vi "Main.vi"(7 "sweep rate, /min":dbl=0.2, 8 "sweep to:":dbl=-0.5, 9 "sweep":T3(radio)=enum."time_sweep") -> ()   [LabVIEW 2017] (continued)
                  n2558 = property on="data" class="Arr (strict)"("Value"=w3368) -> ()  [unwired: 2 in, 2 out]
                }
                frame #8 {
                  # "check if voltage \non 2400 SouceMeter 1\nis to be measured"
                  n2559 = property on="data" class="Arr (strict)"() -> ("Value"=w3380:dbl[])  [unwired: 2 in, 2 out]
                  n2560 = local read "2400 1 meas v"() -> (w3379:bool)
                  n2561 = case shown="True" w3379 {
                    tunnel: w3380 -> [w3382 w3393]
                    tunnel: [w3382 w3392] -> w3381
                    frame False {
                      # "we are not measuring 2400 1, voltage (2400_1_v)"
                    }
                    frame True {
                      # "we are  measuring 2400 1, voltage (2400_1_v)"
                      n2562 = local read "2400 1 addr"() -> (w3387:u8)
                      n2563 = Number To Decimal String(number=w3387) -> (decimal integer string=w3386:string)  [unwired: 1 in]
                      n2564 = GPIB Write(0:w3386, 1:":READ?") -> (6:w3391:errorcluster)  [unwired: 3 in, 1 out]
                      n2565 = GPIB Read(0:w3386, 1:3200, 3:w3391) -> (5:w3384:string)  [unwired: 2 in, 2 out]
                      n2566 = String Subset(string=w3384, length (rest)=13) -> (substring=w3383:string)  [unwired: 1 in]
                      n2567 = Fract/Exp String To Number(string=w3383) -> (number=w3389:dbl)  [unwired: 3 in, 1 out]
                      n2568 = Build Array (concatenate)(w3393, w3389) -> (w3392:dbl[])
                    }
                  }
                  n2569 = property on="data" class="Arr (strict)"("Value"=w3381) -> ()  [unwired: 2 in, 2 out]
                }
                frame #9 {
                  # "check if current \non 2400 SouceMeter 1\nis to be measured"
                  n2570 = property on="data" class="Arr (strict)"() -> ("Value"=w3395:dbl[])  [unwired: 2 in, 2 out]
                  n2571 = local read "2400 1 meas i"() -> (w3394:bool)
                  n2572 = case shown="True" w3394 {
                    tunnel: w3395 -> [w3397 w3409]
                    tunnel: [w3397 w3408] -> w3396
                    frame False {
                      # "we are not measuring 2400 1, current (2400_1_i)"
                    }
                    frame True {
                      # "we are  measuring 2400 1, current (2400_1_i)"
                      n2573 = local read "2400 1 addr"() -> (w3403:u8)
                      n2574 = Number To Decimal String(number=w3403) -> (decimal integer string=w3402:string)  [unwired: 1 in]
                      n2575 = GPIB Write(0:w3402, 1:":READ?") -> (6:w3407:errorcluster)  [unwired: 3 in, 1 out]
                      n2576 = GPIB Read(0:w3402, 1:3200, 3:w3407) -> (5:w3400:string)  [unwired: 2 in, 2 out]
                      n2577 = String Subset(string=w3400, offset (0)=14, length (rest)=13) -> (substring=w3399:string)
                      n2578 = Fract/Exp String To Number(string=w3399) -> (number=w3405:dbl)  [unwired: 3 in, 1 out]
                      n2579 = Build Array (concatenate)(w3409, w3405) -> (w3408:dbl[])
                    }
                  }
                  n2580 = property on="data" class="Arr (strict)"("Value"=w3396) -> ()  [unwired: 2 in, 2 out]
                }
                frame #10 {
                  # "check if voltage \non 2400 SouceMeter 2\nis to be measured"
                  n2581 = property on="data" class="Arr (strict)"() -> ("Value"=w3411:dbl[])  [unwired: 2 in, 2 out]
                  n2582 = local read "2400 2 meas v"() -> (w3410:bool)
                  n2583 = case shown="True" w3410 {
                    tunnel: w3411 -> [w3413 w3424]
                    tunnel: [w3413 w3423] -> w3412
                    frame False {
                      # "we are not measuring 2400 2, voltage (2400_2_v)"
                    }
                    frame True {
                      # "we are  measuring 2400 2, voltage (2400_2_v)"
                      n2584 = local read "2400 2 addr"() -> (w3418:u8)
                      n2585 = Number To Decimal String(number=w3418) -> (decimal integer string=w3417:string)  [unwired: 1 in]
                      n2586 = GPIB Write(0:w3417, 1:":READ?") -> (6:w3422:errorcluster)  [unwired: 3 in, 1 out]
                      n2587 = GPIB Read(0:w3417, 1:3200, 3:w3422) -> (5:w3415:string)  [unwired: 2 in, 2 out]
                      n2588 = String Subset(string=w3415, length (rest)=13) -> (substring=w3414:string)  [unwired: 1 in]
                      n2589 = Fract/Exp String To Number(string=w3414) -> (number=w3420:dbl)  [unwired: 3 in, 1 out]
                      n2590 = Build Array (concatenate)(w3424, w3420) -> (w3423:dbl[])
                    }
                  }
                  n2591 = property on="data" class="Arr (strict)"("Value"=w3412) -> ()  [unwired: 2 in, 2 out]
                }
                frame #11 {
                  # "check if current \non 2400 SouceMeter 2\nis to be measured"
                  n2592 = property on="data" class="Arr (strict)"() -> ("Value"=w3426:dbl[])  [unwired: 2 in, 2 out]
                  n2593 = local read "2400 2 meas i"() -> (w3425:bool)
                  n2594 = case shown="True" w3425 {
                    tunnel: w3426 -> [w3428 w3440]
                    tunnel: [w3428 w3439] -> w3427
                    frame False {
                      # "we are not measuring 2400 2, current (2400_2_i)"
                    }
                    frame True {
                      # "we are  measuring 2400 2, current (2400_2_i)"
                      n2595 = local read "2400 2 addr"() -> (w3434:u8)
                      n2596 = Number To Decimal String(number=w3434) -> (decimal integer string=w3433:string)  [unwired: 1 in]
                      n2597 = GPIB Write(0:w3433, 1:":READ?") -> (6:w3438:errorcluster)  [unwired: 3 in, 1 out]
                      n2598 = GPIB Read(0:w3433, 1:3200, 3:w3438) -> (5:w3431:string)  [unwired: 2 in, 2 out]
                      n2599 = String Subset(string=w3431, offset (0)=14, length (rest)=13) -> (substring=w3430:string)
                      n2600 = Fract/Exp String To Number(string=w3430) -> (number=w3436:dbl)  [unwired: 3 in, 1 out]
                      n2601 = Build Array (concatenate)(w3440, w3436) -> (w3439:dbl[])
                    }
                  }
                  n2602 = property on="data" class="Arr (strict)"("Value"=w3427) -> ()  [unwired: 2 in, 2 out]
                }
                frame #12 {
                  # "check if voltage \non 2400 SouceMeter 3\nis to be measured"
                  n2603 = property on="data" class="Arr (strict)"() -> ("Value"=w3442:dbl[])  [unwired: 2 in, 2 out]
                  n2604 = local read "2400 3 meas v"() -> (w3441:bool)
                  n2605 = case shown="True" w3441 {
                    tunnel: w3442 -> [w3444 w3455]
                    tunnel: [w3444 w3454] -> w3443
                    frame False {
                      # "we are not measuring 2400 3, voltage (2400_3_v)"
                    }
                    frame True {
                      # "we are  measuring 2400 3, voltage (2400_3_v)"
                      n2606 = local read "2400 3 addr"() -> (w3449:u8)
                      n2607 = Number To Decimal String(number=w3449) -> (decimal integer string=w3448:string)  [unwired: 1 in]
                      n2608 = GPIB Write(0:w3448, 1:":READ?") -> (6:w3453:errorcluster)  [unwired: 3 in, 1 out]
                      n2609 = GPIB Read(0:w3448, 1:3200, 3:w3453) -> (5:w3446:string)  [unwired: 2 in, 2 out]
                      n2610 = String Subset(string=w3446, length (rest)=13) -> (substring=w3445:string)  [unwired: 1 in]
                      n2611 = Fract/Exp String To Number(string=w3445) -> (number=w3451:dbl)  [unwired: 3 in, 1 out]
                      n2612 = Build Array (concatenate)(w3455, w3451) -> (w3454:dbl[])
                    }
                  }
                  n2613 = property on="data" class="Arr (strict)"("Value"=w3443) -> ()  [unwired: 2 in, 2 out]
                }
                frame #13 {
                  # "check if current \non 2400 SouceMeter 3\nis to be measured"
                  n2614 = property on="data" class="Arr (strict)"() -> ("Value"=w3457:dbl[])  [unwired: 2 in, 2 out]
                  n2615 = local read "2400 3 meas i"() -> (w3456:bool)
                  n2616 = case shown="True" w3456 {
                    tunnel: w3457 -> [w3459 w3471]
                    tunnel: [w3459 w3470] -> w3458
                    frame False {
                      # "we are not measuring 2400 3, current (2400_3_i)"
                    }
                    frame True {
                      # "we are  measuring 2400 3, current (2400_3_i)"
                      n2617 = local read "2400 3 addr"() -> (w3465:u8)
                      n2618 = Number To Decimal String(number=w3465) -> (decimal integer string=w3464:string)  [unwired: 1 in]
                      n2619 = GPIB Write(0:w3464, 1:":READ?") -> (6:w3469:errorcluster)  [unwired: 3 in, 1 out]
                      n2620 = GPIB Read(0:w3464, 1:3200, 3:w3469) -> (5:w3462:string)  [unwired: 2 in, 2 out]
                      n2621 = String Subset(string=w3462, offset (0)=14, length (rest)=13) -> (substring=w3461:string)
                      n2622 = Fract/Exp String To Number(string=w3461) -> (number=w3467:dbl)  [unwired: 3 in, 1 out]
                      n2623 = Build Array (concatenate)(w3471, w3467) -> (w3470:dbl[])
                    }
                  }
                  n2624 = property on="data" class="Arr (strict)"("Value"=w3458) -> ()  [unwired: 2 in, 2 out]
                }
                frame #14 {
                  # "check if 1st channel \non Keithley 2182A 1\nis to be measured"
                  n2625 = property on="data" class="Arr (strict)"() -> ("Value"=w3473:dbl[])  [unwired: 2 in, 2 out]
                  n2626 = local read "2182A 1 ch1"() -> (w3472:bool)
                  n2627 = case shown="True" w3472 {
                    tunnel: w3473 -> [w3475 w3484]
                    tunnel: [w3475 w3483] -> w3474
                    frame False {
                      # "we are not measuring 2182A 1 channel 1 (2182A_1_ch1)"
                    }
                    frame True {
                      # "we are  measuring 2182A 1 channel 1 (2182A_1_ch1)"
                      n2628 = local read "2182A 1 addr"() -> (w3478:u8)
                      n2629 = Number To Decimal String(number=w3478) -> (decimal integer string=w3477:string)  [unwired: 1 in]
                      n2630 = GPIB Write(0:w3477, 1:":SENSe:DATA:FRES?") -> (6:w3482:errorcluster)  [unwired: 3 in, 1 out]
                      n2631 = GPIB Read(0:w3477, 1:200, 3:w3482) -> (5:w3476:string)  [unwired: 2 in, 2 out]
                      n2632 = Fract/Exp String To Number(string=w3476) -> (number=w3480:dbl)  [unwired: 3 in, 1 out]
                      n2633 = Build Array (concatenate)(w3484, w3480) -> (w3483:dbl[])
                    }
                  }
                  n2634 = property on="data" class="Arr (strict)"("Value"=w3474) -> ()  [unwired: 2 in, 2 out]
                }
                frame #15 {
                  # "check if 2nd channel \non Keithley 2182A 1\nis to be measured"
                  n2635 = property on="data" class="Arr (strict)"() -> ("Value"=w3486:dbl[])  [unwired: 2 in, 2 out]
                  n2636 = local read "2182A 1 ch2"() -> (w3485:bool)
                  n2637 = case shown="True" w3485 {
                    tunnel: w3486 -> [w3488 w3501]
                    tunnel: [w3488 w3500] -> w3487
                    frame False {
                      # "we are not measuring 2182A 1 channel 2 (2182A_1_ch2)"
                    }
                    frame True {
                      # "switching to channel 2 and then\nback to channel 1"
                      # "we are  measuring 2182A 1 channel 2 (2182A_1_ch2)"
                      n2638 = local read "2182A 1 addr"() -> (w3495:u8)
                      n2639 = Number To Decimal String(number=w3495) -> (decimal integer string=w3490:string)  [unwired: 1 in]
                      n2640 = GPIB Write(0:w3490, 1:":SENSe:CHAN 2") -> (6:w3492:errorcluster)  [unwired: 3 in, 1 out]
                      n2641 = GPIB Write(0:w3490, 1:":SENSe:DATA:FRES?", 3:w3492) -> (6:w3499:errorcluster)  [unwired: 2 in, 1 out]
                      n2642 = GPIB Read(0:w3490, 1:200, 3:w3499) -> (5:w3494:string, 7:w3491:errorcluster)  [unwired: 2 in, 1 out]
                      n2643 = GPIB Write(0:w3490, 1:":SENSe:CHAN 1", 3:w3491) -> ()  [unwired: 2 in, 2 out]
                      n2644 = Fract/Exp String To Number(string=w3494) -> (number=w3497:dbl)  [unwired: 3 in, 1 out]
                      n2645 = Build Array (concatenate)(w3501, w3497) -> (w3500:dbl[])
                    }
                  }
                  n2646 = property on="data" class="Arr (strict)"("Value"=w3487) -> ()  [unwired: 2 in, 2 out]
                }
                frame #16 {
                  # "check if 1st channel \non Keithley 2182A 2\nis to be measured"
                  n2647 = property on="data" class="Arr (strict)"() -> ("Value"=w3503:dbl[])  [unwired: 2 in, 2 out]
                  n2648 = local read "2182A 2 ch1"() -> (w3502:bool)
                  n2649 = case shown="True" w3502 {
                    tunnel: w3503 -> [w3505 w3514]
                    tunnel: [w3505 w3513] -> w3504
                    frame False {
                      # "we are not measuring 2182A 2 channel 1 (2182A_2_ch1)"
                    }
                    frame True {
                      # "we are  measuring 2182A 2 channel 1 (2182A_2_ch1)"
                      n2650 = local read "2182A 2 addr"() -> (w3508:u8)
                      n2651 = Number To Decimal String(number=w3508) -> (decimal integer string=w3507:string)  [unwired: 1 in]
                      n2652 = GPIB Write(0:w3507, 1:":SENSe:DATA:FRES?") -> (6:w3512:errorcluster)  [unwired: 3 in, 1 out]
                      n2653 = GPIB Read(0:w3507, 1:200, 3:w3512) -> (5:w3506:string)  [unwired: 2 in, 2 out]
                      n2654 = Fract/Exp String To Number(string=w3506) -> (number=w3510:dbl)  [unwired: 3 in, 1 out]
                      n2655 = Build Array (concatenate)(w3514, w3510) -> (w3513:dbl[])
                    }
                  }
                  n2656 = property on="data" class="Arr (strict)"("Value"=w3504) -> ()  [unwired: 2 in, 2 out]
                }
                frame #17 {
                  # "check if 2nd channel \non Keithley 2182A 2\nis to be measured"
                  n2657 = property on="data" class="Arr (strict)"() -> ("Value"=w3516:dbl[])  [unwired: 2 in, 2 out]
                  n2658 = local read "2182A 2 ch2"() -> (w3515:bool)
                  n2659 = case shown="True" w3515 {
                    tunnel: w3516 -> [w3518 w3531]
                    tunnel: [w3518 w3530] -> w3517
                    frame False {
                      # "we are not measuring 2182A 2 channel 2 (2182A_2_ch2)"
                    }
                    frame True {
                      # "switching to channel 2 and then\nback to channel 1"
                      # "we are  measuring 2182A 2 channel 2 (2182A_2_ch2)"
                      n2660 = local read "2182A 2 addr"() -> (w3525:u8)
                      n2661 = Number To Decimal String(number=w3525) -> (decimal integer string=w3520:string)  [unwired: 1 in]
                      n2662 = GPIB Write(0:w3520, 1:":SENSe:CHAN 2") -> (6:w3522:errorcluster)  [unwired: 3 in, 1 out]
                      n2663 = GPIB Write(0:w3520, 1:":SENSe:DATA:FRES?", 3:w3522) -> (6:w3529:errorcluster)  [unwired: 2 in, 1 out]
                      n2664 = GPIB Read(0:w3520, 1:200, 3:w3529) -> (5:w3524:string, 7:w3521:errorcluster)  [unwired: 2 in, 1 out]
                      n2665 = GPIB Write(0:w3520, 1:":SENSe:CHAN 1", 3:w3521) -> ()  [unwired: 2 in, 2 out]
                      n2666 = Fract/Exp String To Number(string=w3524) -> (number=w3527:dbl)  [unwired: 3 in, 1 out]
                      n2667 = Build Array (concatenate)(w3531, w3527) -> (w3530:dbl[])
                    }
                  }
                  n2668 = property on="data" class="Arr (strict)"("Value"=w3517) -> ()  [unwired: 2 in, 2 out]
                }
                frame #18 {
                  # "check if 1st channel \non Keithley 2182A 3\nis to be measured"
                  n2669 = property on="data" class="Arr (strict)"() -> ("Value"=w3533:dbl[])  [unwired: 2 in, 2 out]
                  n2670 = local read "2182A 3 ch1"() -> (w3532:bool)
                  n2671 = case shown="True" w3532 {
                    tunnel: w3533 -> [w3535 w3544]
                    tunnel: [w3535 w3543] -> w3534
                    frame False {
                      # "we are not measuring 2182A 3 channel 1 (2182A_3_ch1)"
                    }
                    frame True {
                      # "we are  measuring 2182A 3 channel 1 (2182A_3_ch1)"
                      n2672 = local read "2182A 3 addr"() -> (w3538:u8)
                      n2673 = Number To Decimal String(number=w3538) -> (decimal integer string=w3537:string)  [unwired: 1 in]
                      n2674 = GPIB Write(0:w3537, 1:":SENSe:DATA:FRES?") -> (6:w3542:errorcluster)  [unwired: 3 in, 1 out]
                      n2675 = GPIB Read(0:w3537, 1:200, 3:w3542) -> (5:w3536:string)  [unwired: 2 in, 2 out]
                      n2676 = Fract/Exp String To Number(string=w3536) -> (number=w3540:dbl)  [unwired: 3 in, 1 out]
                      n2677 = Build Array (concatenate)(w3544, w3540) -> (w3543:dbl[])
                    }
                  }
                  n2678 = property on="data" class="Arr (strict)"("Value"=w3534) -> ()  [unwired: 2 in, 2 out]
                }
                frame #19 {
                  # "check if 2nd channel \non Keithley 2182A 3\nis to be measured"
                  n2679 = property on="data" class="Arr (strict)"() -> ("Value"=w3546:dbl[])  [unwired: 2 in, 2 out]
                  n2680 = local read "2182A 3 ch2"() -> (w3545:bool)
                  n2681 = case shown="True" w3545 {
                    tunnel: w3546 -> [w3548 w3561]
                    tunnel: [w3548 w3560] -> w3547
                    frame False {
                      # "we are not measuring 2182A 3 channel 2 (2182A_3_ch2)"
                    }
                    frame True {
                      # "switching to channel 2 and then\nback to channel 1"
                      # "we are  measuring 2182A 3 channel 2 (2182A_3_ch2)"
                      n2682 = local read "2182A 3 addr"() -> (w3555:u8)
                      n2683 = Number To Decimal String(number=w3555) -> (decimal integer string=w3550:string)  [unwired: 1 in]
                      n2684 = GPIB Write(0:w3550, 1:":SENSe:CHAN 2") -> (6:w3552:errorcluster)  [unwired: 3 in, 1 out]
                      n2685 = GPIB Write(0:w3550, 1:":SENSe:DATA:FRES?", 3:w3552) -> (6:w3559:errorcluster)  [unwired: 2 in, 1 out]
                      n2686 = GPIB Read(0:w3550, 1:200, 3:w3559) -> (5:w3554:string, 7:w3551:errorcluster)  [unwired: 2 in, 1 out]
                      n2687 = GPIB Write(0:w3550, 1:":SENSe:CHAN 1", 3:w3551) -> ()  [unwired: 2 in, 2 out]
                      n2688 = Fract/Exp String To Number(string=w3554) -> (number=w3557:dbl)  [unwired: 3 in, 1 out]
                      n2689 = Build Array (concatenate)(w3561, w3557) -> (w3560:dbl[])
                    }
                  }
                  n2690 = property on="data" class="Arr (strict)"("Value"=w3547) -> ()  [unwired: 2 in, 2 out]
                }
                frame #20 {
                  # "check if 1st channel \non Keithley 2182A 4\nis to be measured"
                  n2691 = property on="data" class="Arr (strict)"() -> ("Value"=w3563:dbl[])  [unwired: 2 in, 2 out]
                  n2692 = local read "2182A 4 ch1"() -> (w3562:bool)
                  n2693 = case shown="True" w3562 {
                    tunnel: w3563 -> [w3565 w3574]
                    tunnel: [w3565 w3573] -> w3564
                    frame False {
                      # "we are not measuring 2182A 4 channel 1 (2182A_4_ch1)"
                    }
                    frame True {
                      # "we are  measuring 2182A 4 channel 1 (2182A_4_ch1)"
                      n2694 = local read "2182A 4 addr"() -> (w3568:u8)
                      n2695 = Number To Decimal String(number=w3568) -> (decimal integer string=w3567:string)  [unwired: 1 in]
                      n2696 = GPIB Write(0:w3567, 1:":SENSe:DATA:FRES?") -> (6:w3572:errorcluster)  [unwired: 3 in, 1 out]
                      n2697 = GPIB Read(0:w3567, 1:200, 3:w3572) -> (5:w3566:string)  [unwired: 2 in, 2 out]
                      n2698 = Fract/Exp String To Number(string=w3566) -> (number=w3570:dbl)  [unwired: 3 in, 1 out]
                      n2699 = Build Array (concatenate)(w3574, w3570) -> (w3573:dbl[])
                    }
                  }
                  n2700 = property on="data" class="Arr (strict)"("Value"=w3564) -> ()  [unwired: 2 in, 2 out]
                }
                frame #21 {
                  # "check if 2nd channel \non Keithley 2182A 4\nis to be measured"
                  n2701 = property on="data" class="Arr (strict)"() -> ("Value"=w3576:dbl[])  [unwired: 2 in, 2 out]
                  n2702 = local read "2182A 4 ch2"() -> (w3575:bool)
                  n2703 = case shown="False" w3575 {
                    tunnel: w3576 -> [w3578 w3591]
                    tunnel: [w3578 w3590] -> w3577
                    frame False {
                      # "we are not measuring 2182A 4 channel 2 (2182A_4_ch2)"
                    }
                    frame True {
                      # "switching to channel 2 and then\nback to channel 1"
                      # "we are  measuring 2182A 4 channel 2 (2182A_4_ch2)"
                      n2704 = local read "2182A 4 addr"() -> (w3585:u8)
                      n2705 = Number To Decimal String(number=w3585) -> (decimal integer string=w3580:string)  [unwired: 1 in]
                      n2706 = GPIB Write(0:w3580, 1:":SENSe:CHAN 2") -> (6:w3582:errorcluster)  [unwired: 3 in, 1 out]
                      n2707 = GPIB Write(0:w3580, 1:":SENSe:DATA:FRES?", 3:w3582) -> (6:w3589:errorcluster)  [unwired: 2 in, 1 out]
                      n2708 = GPIB Read(0:w3580, 1:200, 3:w3589) -> (5:w3584:string, 7:w3581:errorcluster)  [unwired: 2 in, 1 out]
                      n2709 = GPIB Write(0:w3580, 1:":SENSe:CHAN 1", 3:w3581) -> ()  [unwired: 2 in, 2 out]
                      n2710 = Fract/Exp String To Number(string=w3584) -> (number=w3587:dbl)  [unwired: 3 in, 1 out]
                      n2711 = Build Array (concatenate)(w3591, w3587) -> (w3590:dbl[])
                    }
                  }
                  n2712 = property on="data" class="Arr (strict)"("Value"=w3577) -> ()  [unwired: 2 in, 2 out]
                }
                frame #22 {
                  # "check if voltage on\nKeithley 2636A smua\nis to be measured"
                  n2713 = local read "2636A smua meas v"() -> (w3592:bool)
                  n2714 = property on="data" class="Arr (strict)"() -> ("Value"=w3593:dbl[])  [unwired: 2 in, 2 out]
                  n2715 = case shown="True" w3592 {
                    tunnel: w3593 -> [w3595 w3601]
                    tunnel: [w3595 w3600] -> w3594
                    frame False {
                      # "we are not measuring voltage on 2636A smua (2636A_smua_v)"
                    }
                    frame True {
                      # "we are  measuring voltage on 2636A smua (2636A_smua_v)"
                      n2716 = local read "2336A addr"() -> (w3596:refnum<visa-resource-name>)
                      n2717 = call "SinglePointMeasurement.vi"("Measure"=Measure."Voltage", "Channel"=Channel."a", "VISA resource name 2"=w3596) -> ("Measuremet"=w3598:dbl)  [unwired: 3 in, 4 out]
                      n2718 = Build Array (concatenate)(w3601, w3598) -> (w3600:dbl[])
                    }
                  }
                  n2719 = property on="data" class="Arr (strict)"("Value"=w3594) -> ()  [unwired: 2 in, 2 out]
                }
                frame #23 {
                  # "check if current on\nKeithley 2636A smua\nis to be measured"
                  n2720 = local read "2636A smua meas i"() -> (w3602:bool)
                  n2721 = property on="data" class="Arr (strict)"() -> ("Value"=w3603:dbl[])  [unwired: 2 in, 2 out]
                  n2722 = case shown="True" w3602 {
                    tunnel: w3603 -> [w3605 w3608]
                    tunnel: [w3605 w3607] -> w3604
                    frame False {
                      # "we are not measuring current on 2636A smua (2636A_smua_i)"
                    }
                    frame True {
                      # "we are  measuring current on 2636A smua (2636A_smua_i)"
                      n2723 = stacked-sequence {
                        tunnel: [_ w3617] -> w3606
                        frame #0 {
                          n2724 = local read "auto\nrange A"() -> (w3612:bool)
                          n2725 = local read "2336A addr"() -> (w3615:refnum<visa-resource-name>)
                          n2726 = Select(t="smua.AUTORANGE_ON", s=w3612, f="smua.AUTORANGE_OFF") -> (s? t:f=w3610:string)
                          n2727 = Concatenate Strings("smua.measure.autorangei = ", w3610) -> (w3609:string)
                          n2728 = VISA Write(VISA resource name=w3615, write buffer=w3609) -> ()  [unwired: 1 in, 3 out]
                        }
                        frame #1 {
                          n2729 = local read "2336A addr"() -> (w3619:refnum<visa-resource-name>)
                          n2730 = call "SinglePointMeasurement.vi"("Measure"=Measure."Current", "Channel"=Channel."a", "VISA resource name 2"=w3619) -> ("Measuremet"=w3617:dbl)  [unwired: 3 in, 4 out]
                        }
                      }
                      n2731 = Build Array (concatenate)(w3608, w3606) -> (w3607:dbl[])
                    }
                  }
                  n2732 = property on="data" class="Arr (strict)"("Value"=w3604) -> ()  [unwired: 2 in, 2 out]
                }
                frame #24 {
                  # "check if voltage on\nKeithley 2636A smub\nis to be measured"
                  n2733 = local read "2636A smub meas v"() -> (w3620:bool)
                  n2734 = property on="data" class="Arr (strict)"() -> ("Value"=w3621:dbl[])  [unwired: 2 in, 2 out]
                  n2735 = case shown="True" w3620 {
                    tunnel: w3621 -> [w3623 w3629]
                    tunnel: [w3623 w3628] -> w3622
                    frame False {
                      # "we are not measuring voltage on 2636A smub (2636A_smub_v)"
                    }
                    frame True {
                      # "we are  measuring voltage on 2636A smub (2636A_smub_v)"
                      n2736 = local read "2336A addr"() -> (w3627:refnum<visa-resource-name>)
                      n2737 = call "SinglePointMeasurement.vi"("Measure"=Measure."Voltage", "Channel"=Channel."b", "VISA resource name 2"=w3627) -> ("Measuremet"=w3625:dbl)  [unwired: 3 in, 4 out]
                      n2738 = Build Array (concatenate)(w3629, w3625) -> (w3628:dbl[])
                    }
                  }
                  n2739 = property on="data" class="Arr (strict)"("Value"=w3622) -> ()  [unwired: 2 in, 2 out]
                }
                frame #25 {
                  # "check if current on\nKeithley 2636A smub\nis to be measured"
                  n2740 = local read "2636A smub meas i"() -> (w3630:bool)
                  n2741 = property on="data" class="Arr (strict)"() -> ("Value"=w3631:dbl[])  [unwired: 2 in, 2 out]
                  n2742 = case shown="True" w3630 {
                    tunnel: w3631 -> [w3633 w3636]
                    tunnel: [w3633 w3635] -> w3632
                    frame False {
                      # "we are not measuring current on 2636A smub (2636A_smub_i)"
                    }
                    frame True {
                      # "we are  measuring current on 2636A smub (2636A_smub_i)"
                      n2743 = stacked-sequence {
                        tunnel: [_ w3645] -> w3634
                        frame #0 {
                          n2744 = local read "auto\nrange B"() -> (w3640:bool)
                          n2745 = local read "2336A addr"() -> (w3643:refnum<visa-resource-name>)
                          n2746 = Select(t="smub.AUTORANGE_ON", s=w3640, f="smub.AUTORANGE_OFF") -> (s? t:f=w3638:string)
                          n2747 = Concatenate Strings("smub.measure.autorangei = ", w3638) -> (w3637:string)
                          n2748 = VISA Write(VISA resource name=w3643, write buffer=w3637) -> ()  [unwired: 1 in, 3 out]
                        }
                        frame #1 {
                          n2749 = local read "2336A addr"() -> (w3647:refnum<visa-resource-name>)
                          n2750 = call "SinglePointMeasurement.vi"("Measure"=Measure."Current", "Channel"=Channel."b", "VISA resource name 2"=w3647) -> ("Measuremet"=w3645:dbl)  [unwired: 3 in, 4 out]
                        }
                      }
                      n2751 = Build Array (concatenate)(w3636, w3634) -> (w3635:dbl[])
                    }
                  }
                  n2752 = property on="data" class="Arr (strict)"("Value"=w3632) -> ()  [unwired: 2 in, 2 out]
                }
                frame #26 {
                  # "check if time\nis to be measured"
                  n2753 = property on="data" class="Arr (strict)"() -> ("Value"=w3650:dbl[])  [unwired: 2 in, 2 out]
                  n2754 = local read "measure time"() -> (w3649:bool)
                  n2755 = case shown="True" w3649 {
                    tunnel: w3650 -> [w3652 w3658]
                    tunnel: [w3652 w3657] -> w3651
                    tunnel: w3648 -> [_ w3655]
                    frame False {
                      # "we are not measuring time"
                    }
                    frame True {
                      # "seconds from the beginning of month"
                      # "we are  measuring time"
                      n2756 = call "timeInSeconds.vi"() -> ("Numeric"=w3656:dbl, "current time"=w3653:timestamp)  [unwired: 2 in]
                      n2757 = property on="current time" class="AbsTime (strict)"("Value"=w3653) -> ()  [unwired: 2 in, 2 out]
                      n2758 = Subtract(x=w3656, y=w3655) -> (x-y=w3654:dbl)
                      n2759 = Build Array (concatenate)(w3658, w3654) -> (w3657:dbl[])
                    }
                  }
                  n2760 = property on="data" class="Arr (strict)"("Value"=w3651) -> ()  [unwired: 2 in, 2 out]
                }
                frame #27 {
                  n2761 = local read "iPS_MagnetField"() -> (w3659:bool)
                  n2762 = property on="data" class="Arr (strict)"() -> ("Value"=w3660:dbl[])  [unwired: 2 in, 2 out]
                  n2763 = case shown="True" w3659 {
                    tunnel: w3660 -> [w3662 w3671]
                    tunnel: [w3662 w3670] -> w3661
                    frame False {
                      # "we are not Measuring magnetic field on IPS120-0"
                    }
                    frame True {
                      w3665 = 1
                      # "Measure magnetic field on Teslatron_iPS_Field"
                      n2764 = local read "IPS120-0 addr_sweep"() -> (w3669:u8)
                      n2765 = Number To Decimal String(number=w3669) -> (decimal integer string=w3668:string)  [unwired: 1 in]
                      n2766 = GPIB Write(0:w3668, 1:"R 7", 2:w3665) -> ()  [unwired: 2 in, 2 out]
                      n2767 = GPIB Read(0:w3668, 1:200 ("byte count"), 2:w3665) -> (5:w3667:string)  [unwired: 2 in, 2 out]
                      n2768 = Fract/Exp String To Number(string=w3667, offset=w3665) -> (number=w3663:dbl)  [unwired: 2 in, 1 out]
                      n2769 = Build Array (concatenate)(w3671, w3663) -> (w3670:dbl[])
                    }
                  }
                  n2770 = property on="data" class="Arr (strict)"("Value"=w3661) -> ()  [unwired: 2 in, 2 out]
                }
                frame #28 {
                  # "check if current \non 2461 SouceMeter\nis to be measured"
                  n2771 = property on="data" class="Arr (strict)"() -> ("Value"=w3673:dbl[])  [unwired: 2 in, 2 out]
                  n2772 = property on="iTC_Sample_T" class="Bool (strict)"() -> ("Value"=w3672:bool)  [unwired: 2 in, 2 out]
                  n2773 = case shown="True" w3672 {
                    tunnel: w3673 -> [w3675 w3688]
                    tunnel: [w3675 w3687] -> w3674
                    frame False {
                      # "we are not measuring 2461, voltage (2461_meas_v)"
                    }
                    frame True {
                      w3676 = 1
                      # "temporarily ITC503S"
                      # "we are  measuring 2461, voltage (2461_meas_v)"
                      n2774 = property on="iTC_503_addr_sweep" class="DigNum (strict)"() -> ("Value"=w3682:u8)  [unwired: 2 in, 2 out]
                      n2775 = Number To Decimal String(number=w3682) -> (decimal integer string=w3683:string)  [unwired: 1 in]
                      n2776 = GPIB Write(0:w3683, 1:"$C3", 2:1) -> (6:w3684:errorcluster)  [unwired: 2 in, 1 out]
                      n2777 = GPIB Write(0:w3683, 1:"R3", 2:w3676, 3:w3684) -> (6:w3686:errorcluster)  [unwired: 1 in, 1 out]
                      n2778 = GPIB Read(0:w3683, 1:200, 2:w3676, 3:w3686) -> (5:w3685:string)  [unwired: 1 in, 2 out]
                      n2779 = Fract/Exp String To Number(string=w3685, offset=w3676) -> (number=w3677:dbl)  [unwired: 2 in, 1 out]
                      n2780 = Build Array (concatenate)(w3688, w3677) -> (w3687:dbl[])
                    }
                  }
                  n2781 = property on="data" class="Arr (strict)"("Value"=w3674) -> ()  [unwired: 2 in, 2 out]
                }
                frame #29 {
                  # "check if current \non 2461 SouceMeter\nis to be measured"
                  n2782 = property on="data" class="Arr (strict)"() -> ("Value"=w3690:dbl[])  [unwired: 2 in, 2 out]
                  n2783 = property on="CH_A" class="Bool (strict)"() -> ("Value"=w3689:bool)  [unwired: 2 in, 2 out]
                  n2784 = case shown="True" w3689 {
                    tunnel: w3690 -> [w3692 w3705]
                    tunnel: [w3692 w3704] -> w3691
                    frame False {
                      # "we are not measuring 2461, voltage (2461_meas_v)"
                    }
                    frame True {
                      w3693 = 1
                      # "temporarily ITC503S"
                      # "we are  measuring 2461, voltage (2461_meas_v)"
                      n2785 = property on="iTC_503_addr_sweep" class="DigNum (strict)"() -> ("Value"=w3699:u8)  [unwired: 2 in, 2 out]
                      n2786 = Number To Decimal String(number=w3699) -> (decimal integer string=w3700:string)  [unwired: 1 in]
                      n2787 = GPIB Write(0:w3700, 1:"$C3", 2:1) -> (6:w3701:errorcluster)  [unwired: 2 in, 1 out]
                      n2788 = GPIB Write(0:w3700, 1:"R3", 2:w3693, 3:w3701) -> (6:w3703:errorcluster)  [unwired: 1 in, 1 out]
                      n2789 = GPIB Read(0:w3700, 1:200, 2:w3693, 3:w3703) -> (5:w3702:string)  [unwired: 1 in, 2 out]
                      n2790 = Fract/Exp String To Number(string=w3702, offset=w3693) -> (number=w3694:dbl)  [unwired: 2 in, 1 out]
                      n2791 = Build Array (concatenate)(w3705, w3694) -> (w3704:dbl[])
                    }
                  }
                  n2792 = property on="data" class="Arr (strict)"("Value"=w3691) -> ()  [unwired: 2 in, 2 out]
                }
                frame #30 {
                  # "check if current \non 2461 SouceMeter\nis to be measured"
                  n2793 = property on="CH_B" class="Bool (strict)"() -> ("Value"=w3706:bool)  [unwired: 2 in, 2 out]
                  n2794 = property on="data" class="Arr (strict)"() -> ("Value"=w3707:dbl[])  [unwired: 2 in, 2 out]
                  n2795 = case shown="True" w3706 {
                    tunnel: w3707 -> [w3709 w3722]
                    tunnel: [w3709 w3721] -> w3708
                    frame False {
                      # "we are not measuring 2461, voltage (2461_meas_v)"
                    }
                    frame True {
                      w3710 = 1
                      # "temporarily ITC503S"
                      # "we are  measuring 2461, voltage (2461_meas_v)"
                      n2796 = property on="iTC_503_addr_sweep" class="DigNum (strict)"() -> ("Value"=w3716:u8)  [unwired: 2 in, 2 out]
                      n2797 = Number To Decimal String(number=w3716) -> (decimal integer string=w3717:string)  [unwired: 1 in]
                      n2798 = GPIB Write(0:w3717, 1:"$C3", 2:1) -> (6:w3718:errorcluster)  [unwired: 2 in, 1 out]
                      n2799 = GPIB Write(0:w3717, 1:"R2", 2:w3710, 3:w3718) -> (6:w3720:errorcluster)  [unwired: 1 in, 1 out]
                      n2800 = GPIB Read(0:w3717, 1:200, 2:w3710, 3:w3720) -> (5:w3719:string)  [unwired: 1 in, 2 out]
                      n2801 = Fract/Exp String To Number(string=w3719, offset=w3710) -> (number=w3711:dbl)  [unwired: 2 in, 1 out]
                      n2802 = Build Array (concatenate)(w3722, w3711) -> (w3721:dbl[])
                    }
                  }
                  n2803 = property on="data" class="Arr (strict)"("Value"=w3708) -> ()  [unwired: 2 in, 2 out]
                }
              }
            }
            frame #4 {
              n2804 = property on="data" class="Arr (strict)"() -> ("Value"=w3723:dbl[])  [unwired: 2 in, 2 out]
            }
          }
          n2805 = stacked-sequence "add data to array" {
            tunnel: w3165 -> [w3177]
            tunnel: [w3176] -> w3164
            tunnel: w3163 -> [w3175]
            frame #0 {
              n2806 = Build Array (concatenate)(w3177, w3175) -> (w3176:dbl[][])
            }
          }
          n2807 = stacked-sequence "plot selected measurements" {
            seq-local: [_ w3200 _] -> [_ _ w3245]
            seq-local: [_ w3199 _] -> [_ _ w3246]
            tunnel: w3164 -> [_ w3198 _]
            frame #0 {
              n2808 = property on="XY Graph" class="XYGraph (strict)"("ActYScl"=0 ("Active Y Scale")) -> (error out=w3183:errorcluster)  [unwired: 2 in, 1 out]
              n2809 = property on="Show cursor" class="Bool (strict)"() -> ("Value"=w3178:bool)  [unwired: 2 in, 2 out]
              n2810 = property on="Xaxis" class="Ring (strict)"() -> ("Value"=w3188:u16)  [unwired: 2 in, 2 out]
              n2811 = property on="Yaxis" class="Ring (strict)"(error in=w3183) -> (error out=w3182:errorcluster, "RingText.Text"=w3181:string)  [unwired: 1 in, 1 out]
              n2812 = property on="XY Graph" class="XYGraph (strict)"("Cursor.Visible"=w3178) -> ()  [unwired: 2 in, 2 out]
              n2813 = property on="Figure_axis" class="Arr (strict)"() -> ("Value"=w3189:string[])  [unwired: 2 in, 2 out]
              n2814 = property on="XY Graph" class="XYGraph (strict)"(error in=w3182, "YScale.NameLbl.Text"=w3181) -> (error out=w3179:errorcluster)  [unwired: 1 in, 1 out]
              n2815 = property on="XY Graph" class="XYGraph (strict)"(error in=w3179, "ActYScl"=1 ("Active Y Scale")) -> (error out=w3185:errorcluster)  [unwired: 1 in, 1 out]
              n2816 = property on="Yright" class="Ring (strict)"(error in=w3185) -> (error out=w3186:errorcluster, "RingText.Text"=w3180:string)  [unwired: 1 in, 1 out]
              n2817 = Index Array(array=w3189, index=w3188) -> (element=w3190:string)
              n2818 = property on="XY Graph" class="XYGraph (strict)"("XScale.NameLbl.Text"=w3190) -> ()  [unwired: 2 in, 2 out]
              n2819 = property on="XY Graph" class="XYGraph (strict)"(error in=w3186, "YScale.NameLbl.Text"=w3180) -> ()  [unwired: 1 in, 2 out]
            }
            frame #1 {
              n2820 = local read "Xaxis"() -> (w3203:u16)
              n2821 = property on="Yright" class="Ring (strict)"() -> ("Value"=w3197:u16)  [unwired: 2 in, 2 out]
              n2822 = property on="Yright" class="Ring (strict)"() -> ("RingText.Text"=w3196:string)  [unwired: 2 in, 2 out]
              n2823 = property on="Xaxis" class="Ring (strict)"() -> ("RingText.Text"=w3202:string)  [unwired: 2 in, 2 out]
              n2824 = property on="Yaxis" class="Ring (strict)"() -> ("RingText.Text"=w3201:string)  [unwired: 2 in, 2 out]
              n2825 = local read "Yaxis"() -> (w3204:u16)
              n2826 = case shown="\"formula\"" w3196 {
                tunnel: [w3209 w3216] -> w3194
                tunnel: w3197 -> [_ w3215]
                tunnel: w3198 -> [w3210 w3214]
                tunnel: [w3208 errorcluster {"status"=FALSE, "code"=0, "source"=""} ("error out")] -> _
                frame "formula" {
                  n2827 = local read "formula_variables"() -> (w3211:string[])
                  n2828 = Transpose 2D Array(2D array=w3210) -> (transposed array=w3212:dbl[][])
                  n2829 = property on="Y_right_formula" class="Str"() -> ("Value"=w3207:string)  [unwired: 2 in, 2 out]
                  n2830 = call <vilib>:"Eval Multi-Variable Array.vi"("Variables"=w3211, "X Values"=w3212, "formula"=w3207) -> ("error out"=w3208:errorcluster, "Y Values"=w3209:dbl[])  [unwired: 1 in]
                }
                frame "0", Default {
                  n2831 = Index Array(array=w3214, index (col)=w3215) -> (element=w3216:dbl[])  [unwired: 1 in]
                }
              }
              n2832 = case shown="\"formula\"" w3202 {
                tunnel: [w3227 w3232] -> w3206
                tunnel: w3203 -> [w3230 _]
                tunnel: w3198 -> [w3229 w3236]
                tunnel: [errorcluster {"status"=FALSE, "code"=0, "source"=""} ("error out") w3233] -> w3200
                tunnel: [w3227 w3232] -> w3195
                frame "0", Default {
                  n2833 = Index Array(array=w3229, index (col)=w3230) -> (element=w3227:dbl[])  [unwired: 1 in]
                }
                frame "formula" {
                  n2834 = local read "formula_variables"() -> (w3235:string[])
                  n2835 = Transpose 2D Array(2D array=w3236) -> (transposed array=w3234:dbl[][])
                  n2836 = property on="X_axis_formula" class="Str"() -> ("Value"=w3231:string)  [unwired: 2 in, 2 out]
                  n2837 = call <vilib>:"Eval Multi-Variable Array.vi"("Variables"=w3235, "X Values"=w3234, "formula"=w3231) -> ("error out"=w3233:errorcluster, "Y Values"=w3232:dbl[])  [unwired: 1 in]
                }
              }
              n2838 = case shown="\"formula\"" w3201 {
                tunnel: [w3219 w3226] -> w3205
                tunnel: w3204 -> [_ w3225]
                tunnel: w3198 -> [w3220 w3224]
                tunnel: [w3218 errorcluster {"status"=FALSE, "code"=0, "source"=""} ("error out")] -> w3199
                frame "formula" {
                  n2839 = local read "formula_variables"() -> (w3221:string[])
                  n2840 = Transpose 2D Array(2D array=w3220) -> (transposed array=w3222:dbl[][])
                  n2841 = property on="Y_left_formula" class="Str"() -> ("Value"=w3217:string)  [unwired: 2 in, 2 out]
                  n2842 = call <vilib>:"Eval Multi-Variable Array.vi"("Variables"=w3221, "X Values"=w3222, "formula"=w3217) -> ("error out"=w3218:errorcluster, "Y Values"=w3219:dbl[])  [unwired: 1 in]
                }
                frame "0", Default {
                  n2843 = Index Array(array=w3224, index (col)=w3225) -> (element=w3226:dbl[])  [unwired: 1 in]
                }
              }
              n2844 = Bundle("Y Values"=w3206, "Y Values"=w3205) -> (w3193:cluster{"Y Values":dbl[], "Y Values":dbl[]})  [unwired: 1 in]
              n2845 = Bundle("Y Values"=w3195, "Y Values"=w3194) -> (w3192:cluster{"Y Values":dbl[], "Y Values":dbl[]})  [unwired: 1 in]
              n2846 = Build Array(w3193, w3192) -> (w3191:cluster{"Y Values":dbl[], "Y Values":dbl[]}[])
              n2847 = property on="XY Graph" class="XYGraph (strict)"("Value"=w3191) -> ()  [unwired: 2 in, 2 out]
            }
            frame #2 {
              # "show if formula \nis wrong"
              n2848 = property on="Yaxis" class="Ring (strict)"() -> ("RingText.Text"=w3242:string)  [unwired: 2 in, 2 out]
              n2849 = property on="XY Graph" class="XYGraph (strict)"("Active Plot"=u32 0, "Plot.Plot Name"=w3242) -> (error out=w3243:errorcluster)  [unwired: 2 in, 1 out]
              n2850 = property on="Yright" class="Ring (strict)"() -> ("RingText.Text"=w3240:string)  [unwired: 2 in, 2 out]
              n2851 = property on="XY Graph" class="XYGraph (strict)"(error in=w3243, "Active Plot"=u32 1, "Plot.Plot Name"=w3240) -> ()  [unwired: 1 in, 2 out]
              n2852 = Unbundle By Name(w3246) -> ("status"=w3239:bool)
              n2853 = Unbundle By Name(w3245) -> ("status"=w3238:bool)
              n2854 = Unbundle By Name(w3245) -> ("status"=w3237:bool)
              n2855 = property on="status 3" class="Bool (strict)"("Value"=w3237) -> ()  [unwired: 2 in, 2 out]
              n2856 = property on="status 2" class="Bool (strict)"("Value"=w3239) -> ()  [unwired: 2 in, 2 out]
              n2857 = property on="status" class="Bool (strict)"("Value"=w3238) -> ()  [unwired: 2 in, 2 out]
            }
          }
          n2858 = stacked-sequence "set next value in the sweep" {
            tunnel: w3174 -> [w3724 _]
            tunnel: [w3724 _] -> w3173
            tunnel: w3171 -> [_ w3846]
            tunnel: w3169 -> [w3728 _]
            frame #0 {
              n2859 = local read "sweep"() -> (w3731:T3)
              n2860 = property on="Sweep Channel" class="DigNum (strict)"("Value"=w3724) -> ()  [unwired: 2 in, 2 out]
              n2861 = property on="sweep value" class="DigNum (strict)"("Value"=w3724) -> ()  [unwired: 2 in, 2 out]
              n2862 = case shown="\"2400_1\"" w3731 {
                tunnel: w3724 -> [w3744 w3752 w3758 w3767 w3789 _ w3790 w3813]
                tunnel: w3728 -> [_ _ _ w3766 _ _ _ _]
                frame "2400_1" {
                  # "sweep voltage on 2400 1"
                  n2863 = local read "2400 1 addr"() -> (w3746:u8)
                  n2864 = Number To Fractional String(number=w3744) -> (F-format string=w3750:string)  [unwired: 3 in]
                  n2865 = Concatenate Strings(":INIT:IMM; :SOUR:VOLT:LEV:IMM:AMPL " ("data"), w3750) -> (w3748:string)
                  n2866 = Number To Decimal String(number=w3746) -> (decimal integer string=w3745:string)  [unwired: 1 in]
                  n2867 = GPIB Write(0:w3745, 1:w3748, 2:i16 1 ("mode (0)")) -> ()  [unwired: 2 in, 2 out]
                }
                frame "2400_2" {
                  # "sweep curr on 2400 2"
                  n2868 = Number To Fractional String(number=w3752) -> (F-format string=w3757:string)  [unwired: 3 in]
                  n2869 = local read "2400 2 addr"() -> (w3754:u8)
                  n2870 = Concatenate Strings(":INIT:IMM; :SOUR:CURR:LEV:IMM:AMPL " ("data"), w3757) -> (w3755:string)
                  n2871 = Number To Decimal String(number=w3754) -> (decimal integer string=w3753:string)  [unwired: 1 in]
                  n2872 = GPIB Write(0:w3753, 1:w3755, 2:i16 1 ("mode (0)")) -> ()  [unwired: 2 in, 2 out]
                }
                frame "2400_3" {
                  # "sweep voltage on 2400 3"
                  n2873 = local read "2400 3 addr"() -> (w3760:u8)
                  n2874 = Number To Fractional String(number=w3758) -> (F-format string=w3764:string)  [unwired: 3 in]
                  n2875 = Concatenate Strings(":INIT:IMM; :SOUR:VOLT:LEV:IMM:AMPL " ("data"), w3764) -> (w3762:string)
                  n2876 = Number To Decimal String(number=w3760) -> (decimal integer string=w3759:string)  [unwired: 1 in]
                  n2877 = GPIB Write(0:w3759, 1:w3762, 2:i16 1 ("mode (0)")) -> ()  [unwired: 2 in, 2 out]
                }
                frame "2636a_smua" {
                  n2878 = property on="sweep" class="Bool (strict)"() -> ("Value"=w3765:bool)  [unwired: 2 in, 2 out]
                  n2879 = case shown="False" w3765 {
                    tunnel: w3767 -> [w3772 w3785]
                    tunnel: w3766 -> [w3769 _]
                    frame True {
                      w3770 = 30.0 ("y")
                      n2880 = Subtract(x=w3772, y=w3769) -> (x-y=w3771:dbl)
                      n2881 = Divide(x=w3771, y=w3770) -> (x/y=w3768:dbl)
                      n2882 = for {
                        N: w3770 -> [_]
                        tunnel: w3769 -> [w3778]
                        tunnel: w3768 -> [w3776]
                        i -> [w3777]
                        n2883 = Multiply(x=w3776, y=w3777) -> (x*y=w3775:dbl)
                        n2884 = local read "2336A addr"() -> (w3780:refnum<visa-resource-name>)
                        n2885 = Add(x=w3775, y=w3778) -> (x+y=w3774:dbl)
                        n2886 = call "setLevel.vi"("VISA resource name 2"=w3780, "Source"=Source."Voltage", "Channel"=Channel."a", "SourceLevel"=w3774) -> ()  [unwired: 1 in, 3 out]
                        n2887 = Wait (ms)(milliseconds to wait=u32 12) -> ()  [unwired: 1 out]
                      }
                    }
                    frame False {
                      # "sweep voltage on 2636a smua"
                      n2888 = local read "2336A addr"() -> (w3783:refnum<visa-resource-name>)
                      n2889 = call "setLevel.vi"("VISA resource name 2"=w3783, "Source"=Source."Voltage", "Channel"=Channel."a", "SourceLevel"=w3785) -> ()  [unwired: 1 in, 3 out]
                    }
                  }
                }
                frame "2636a_smub" {
                  # "sweep voltage on 2636b smua"
                  n2890 = local read "2336A addr"() -> (w3786:refnum<visa-resource-name>)
                  n2891 = call "setLevel.vi"("VISA resource name 2"=w3786, "Source"=Source."Voltage", "Channel"=Channel."b", "SourceLevel"=w3789) -> ()  [unwired: 1 in, 3 out]
                }
                frame "time_sweep", Default {
                  # "do not sweep, just time"
                }
                frame "iPS" {
                  n2892 = stacked-sequence {
                    tunnel: w3790 -> [_ _ _ _ w3804 _ _]
                    frame #0 {
                      n2893 = local read "IPS120-0 addr_sweep"() -> (w3794:u8)
                      n2894 = Number To Decimal String(number=w3794) -> (decimal integer string=w3793:string)  [unwired: 1 in]
                      n2895 = GPIB Write(0:w3793, 1:"$C3", 2:i16 1 ("mode (0)")) -> ()  [unwired: 2 in, 2 out]
                    }
                    frame #1 {
                      n2896 = Wait (ms)(milliseconds to wait=u32 100) -> ()  [unwired: 1 out]
                    }
                    frame #2 {
                      n2897 = local read "IPS120-0 addr_sweep"() -> (w3799:u8)
                      n2898 = Number To Decimal String(number=w3799) -> (decimal integer string=w3798:string)  [unwired: 1 in]
                      n2899 = GPIB Write(0:w3798, 1:"$A1", 2:i16 1 ("mode (0)")) -> ()  [unwired: 2 in, 2 out]
                    }
                    frame #3 {
                      n2900 = Wait (ms)(milliseconds to wait=u32 100) -> ()  [unwired: 1 out]
                    }
                    frame #4 {
                      n2901 = Number To Fractional String(number=w3804) -> (F-format string=w3802:string)  [unwired: 3 in]
                      n2902 = local read "IPS120-0 addr_sweep"() -> (w3807:u8)
                      n2903 = Concatenate Strings("$J", w3802) -> (w3803:string)
                      n2904 = Number To Decimal String(number=w3807) -> (decimal integer string=w3806:string)  [unwired: 1 in]
                      n2905 = GPIB Write(0:w3806, 1:w3803, 2:i16 1 ("mode (0)")) -> ()  [unwired: 2 in, 2 out]
                    }
                    frame #5 {
                      n2906 = Wait (ms)(milliseconds to wait=u32 100) -> ()  [unwired: 1 out]
                    }
                    frame #6 {
                      n2907 = local read "IPS120-0 addr_sweep"() -> (w3812:u8)
                      n2908 = Number To Decimal String(number=w3812) -> (decimal integer string=w3811:string)  [unwired: 1 in]
                      n2909 = GPIB Write(0:w3811, 1:"$C2", 2:i16 1 ("mode (0)")) -> ()  [unwired: 2 in, 2 out]
                    }
                  }
                }
                frame "iTC" {
                  n2910 = stacked-sequence {
                    tunnel: w3813 -> [w3823 w3826]
                    frame #0 {
                      n2911 = property on="iTC_503_addr_sweep" class="DigNum (strict)"() -> ("Value"=w3814:u8)  [unwired: 2 in, 2 out]
                      n2912 = Less Or Equal To 0?(x=w3823) -> (x <= 0?=w3825:bool)
                      n2913 = Select(t=0.0, s=w3825, f=w3823) -> (s? t:f=w3815:dbl)
                      n2914 = Number To Decimal String(number=w3814) -> (decimal integer string=w3820:string)  [unwired: 1 in]
                      n2915 = Number To Fractional String(number=w3815, width (-)=5, precision (6)=4) -> (F-format string=w3822:string)  [unwired: 1 in]
                      n2916 = Concatenate Strings("$T ", w3822) -> (w3821:string)
                      n2917 = GPIB Write(0:w3820, 1:w3821, 2:3) -> ()  [unwired: 2 in, 2 out]
                    }
                    frame #1 {
                      n2918 = while {
                        tunnel: w3826 -> [w3839]
                        stop <- w3840 stop-if-true
                        w3831 = 1
                        n2919 = property on="iTC_503_addr_sweep" class="DigNum (strict)"() -> ("Value"=w3827:u8)  [unwired: 2 in, 2 out]
                        n2920 = Number To Decimal String(number=w3827) -> (decimal integer string=w3837:string)  [unwired: 1 in]
                        n2921 = GPIB Write(0:w3837, 1:"$C3", 2:1) -> (6:w3836:errorcluster)  [unwired: 2 in, 1 out]
                        n2922 = GPIB Write(0:w3837, 1:"R3", 2:w3831, 3:w3836) -> (6:w3834:errorcluster)  [unwired: 1 in, 1 out]
                        n2923 = GPIB Read(0:w3837, 1:200, 2:w3831, 3:w3834) -> (5:w3835:string)  [unwired: 1 in, 2 out]
                        n2924 = property on="Tolerance_Sweep" class="DigNum (strict)"() -> ("Value"=w3838:dbl)  [unwired: 2 in, 2 out]
                        n2925 = Fract/Exp String To Number(string=w3835, offset=w3831) -> (number=w3828:dbl)  [unwired: 2 in, 1 out]
                        n2926 = Subtract(x=w3828, y=w3839) -> (x-y=w3842:dbl)
                        n2927 = Absolute Value(x=w3842) -> (abs(x)=w3841:dbl)
                        n2928 = Less?(x=w3841, y=w3838) -> (x < y?=w3840:bool)
                      }
                    }
                  }
                }
              }
              n2929 = property on="Offset" class="DigNum (strict)"() -> ("Value"=w3727:dbl)  [unwired: 2 in, 2 out]
              n2930 = property on="Slope" class="DigNum (strict)"() -> ("Value"=w3726:dbl)  [unwired: 2 in, 2 out]
              n2931 = Multiply(x=w3726, y=w3724) -> (x*y=w3729:dbl)
              n2932 = property on="Double Sweep" class="Bool (strict)"() -> ("Value"=w3725:bool)  [unwired: 2 in, 2 out]
              n2933 = Add(x=w3727, y=w3729) -> (x+y=w3730:dbl)
              n2934 = case shown="False" w3725 {
                tunnel: w3730 -> [_ w3732]
                frame False {
                }
                frame True {
                  n2935 = disable-structure shown="Enabled" {
                    disable-tunnel: w3732 -> [w3733 w3741]
                    frame Disabled {
                      # "sweep voltage on 2400 2"
                      n2936 = local read "2400 2 addr"() -> (w3734:u8)
                      n2937 = Number To Fractional String(number=w3733) -> (F-format string=w3735:string)  [unwired: 3 in]
                      n2938 = Concatenate Strings(":INIT:IMM; :SOUR:VOLT:LEV:IMM:AMPL " ("data"), w3735) -> (w3737:string)
                      n2939 = Number To Decimal String(number=w3734) -> (decimal integer string=w3738:string)  [unwired: 1 in]
                      n2940 = GPIB Write(0:w3738, 1:w3737, 2:i16 1 ("mode (0)")) -> ()  [unwired: 2 in, 2 out]
                    }
                    frame Enabled {
                      n2941 = property on="Slave Channel" class="Enum (strict)"() -> ("Value"=w3740:T1)  [unwired: 2 in, 2 out]
                      n2942 = local read "2336A addr"() -> (w3743:refnum<visa-resource-name>)
                      n2943 = call "setLevel.vi"("VISA resource name 2"=w3743, "Source"=Source."Voltage", "Channel"=w3740, "SourceLevel"=w3741) -> ()  [unwired: 1 in, 3 out]
                    }
                  }
                }
              }
            }
            frame #1 {
              # "calculate deliberate time delay for the next step"
              n2944 = Tick Count (ms)() -> (millisecond timer value=w3848:u32)
              n2945 = Subtract(x=w3848, y=w3846) -> (x-y=w3847:u32)
              n2946 = property on="time/point, sec" class="DigNum (strict)"() -> ("Value"=w3843:dbl)  [unwired: 2 in, 2 out]
              n2947 = Multiply(x=w3843, y=1000.0) -> (x*y=w3845:dbl)
              n2948 = Subtract(x=w3845, y=w3847) -> (x-y=w3844:dbl)
              n2949 = property on="time delay, ms" class="DigNum (strict)"("Value"=w3844) -> ()  [unwired: 2 in, 2 out]
            }
          }
          n2950 = Or(x=w3167, y="Stop Ramp") -> (x .or. y?=w3168:bool)
        }
        n2951 = stacked-sequence {
          tunnel: w2571 -> [_ _]
          tunnel: w2570 -> [_ w3151]
          frame #0 {
            n2952 = stacked-sequence {
              frame #0 {
                n2953 = local read "2636A smua meas v"() -> (w3149:bool)
                n2954 = local read "2636A smub meas v"() -> (w3147:bool)
                n2955 = local read "2636A smub meas i"() -> (w3146:bool)
                n2956 = local read "2636A smua meas i"() -> (w3148:bool)
                n2957 = Compound Arithmetic op=OR(w3149, w3148, w3147, w3146) -> (w3145:bool)
                n2958 = case shown="False" w3145 {
                  frame False {
                  }
                  frame True {
                    # "close session on 2636A"
                    n2959 = local read "2336A addr"() -> (w3150:refnum<visa-resource-name>)
                    n2960 = VISA Close(VISA resource name=w3150) -> ()  [unwired: 1 in, 1 out]
                  }
                }
              }
            }
            n2961 = property on="Stop Ramp" class="Bool"("DisabledEnum"=T5."Disabled and Grayed Out" ("Disabled")) -> ()  [unwired: 2 in, 2 out]
          }
          frame #1 {
            n2962 = property on="Linetrace or Mapping?" class="Bool (strict)"() -> ("Value"=w3152:bool)  [unwired: 2 in, 2 out]
            n2963 = case shown="True" w3152 {
              tunnel: w3151 -> [w3156 w3157]
              frame False {
                w3154 = T5."Enabled" ("Disabled")
                n2964 = Enqueue Element(queue=w3156, element="Idle") -> ()  [unwired: 2 in, 3 out]
                n2965 = property on="sweep" class="RadioBtnsControl (strict)"("DisabledEnum"=w3154) -> ()  [unwired: 2 in, 2 out]
                n2966 = property on="2182A 1 addr" class="DigNum (strict)"("DisabledEnum"=w3154) -> ()  [unwired: 2 in, 2 out]
                n2967 = property on="2182A 2 addr" class="DigNum (strict)"("DisabledEnum"=w3154) -> ()  [unwired: 2 in, 2 out]
                n2968 = property on="2182A 3 addr" class="DigNum (strict)"("DisabledEnum"=w3154) -> ()  [unwired: 2 in, 2 out]
                n2969 = property on="2182A 4 addr" class="DigNum (strict)"("DisabledEnum"=w3154) -> ()  [unwired: 2 in, 2 out]
                n2970 = property on="2400 1 addr" class="DigNum (strict)"("DisabledEnum"=w3154) -> ()  [unwired: 2 in, 2 out]
                n2971 = property on="Sweep Down" class="Bool"("DisabledEnum"=w3154) -> ()  [unwired: 2 in, 2 out]
                n2972 = property on="2400 2 addr" class="DigNum (strict)"("DisabledEnum"=w3154) -> ()  [unwired: 2 in, 2 out]
                n2973 = property on="2400 3 addr" class="DigNum (strict)"("DisabledEnum"=w3154) -> ()  [unwired: 2 in, 2 out]
                n2974 = property on="2336A addr" class="VISAName"("DisabledEnum"=w3154) -> ()  [unwired: 2 in, 2 out]
                n2975 = property on="SR830 1 addr" class="DigNum (strict)"("DisabledEnum"=w3154) -> ()  [unwired: 2 in, 2 out]
                n2976 = property on="SR830 2 addr" class="DigNum (strict)"("DisabledEnum"=w3154) -> ()  [unwired: 2 in, 2 out]
                n2977 = property on="SR830 3 addr" class="DigNum (strict)"("DisabledEnum"=w3154) -> ()  [unwired: 2 in, 2 out]
                n2978 = property on="SR830 4 addr" class="DigNum (strict)"("DisabledEnum"=w3154) -> ()  [unwired: 2 in, 2 out]
                n2979 = property on="Stop Ramp" class="Bool"("DisabledEnum"=T5."Disabled and Grayed Out" ("Disabled")) -> ()  [unwired: 2 in, 2 out]
              }
              frame True {
                n2980 = stacked-sequence {
                  tunnel: w3157 -> [_ w3162]
                  frame #0 {
                    n2981 = property on="Up Rate" class="DigNum (strict)" props=["Value"]() -> ()  [unwired: 2 in, 3 out]
                    n2982 = property on="upper limit" class="DigNum (strict)" props=["Value"]() -> ()  [unwired: 2 in, 3 out]
                    n2983 = property on="Down Rate" class="DigNum (strict)"() -> ("Value"=w3158:dbl)  [unwired: 2 in, 2 out]
                    n2984 = property on="lower limit" class="DigNum (strict)"() -> ("Value"=w3159:dbl)  [unwired: 2 in, 2 out]
                    n2985 = property on="Sweep Direction" class="Str"("Value"="Sweep Down" ("Sweep Direction")) -> ()  [unwired: 2 in, 2 out]
                    n2986 = property on="sweep to:" class="DigNum (strict)"("Value"=w3159) -> ()  [unwired: 2 in, 2 out]
                    n2987 = property on="sweep rate, /min" class="DigNum (strict)"("Value"=w3158) -> ()  [unwired: 2 in, 2 out]
                  }
                  frame #1 {
                    n2988 = Enqueue Element(queue=w3162, element="Step to Next Value") -> ()  [unwired: 2 in, 3 out]
                  }
                }
              }
            }
          }
        }
      }
      frame "Step to Next Value" {
        n2989 = property on="Table Index" class="DigNum (strict)"() -> ("Value"=w3864:dbl)  [unwired: 2 in, 2 out]
        n2990 = property on="Step values" class="Tbl (strict)"() -> ("Value"=w3863:string[][])  [unwired: 2 in, 2 out]
        n2991 = Equal?(x=w3864, y=0) -> (x = y?=w3860:bool)
        n2992 = case shown="False" w3860 {
          tunnel: w3864 -> [w3870 w3876]
          tunnel: cluster{"Row":i32, "Column":i32} {"Row"=0, "Column"=0} ("Active Cell:Active Cell") -> [w3867 w3874]
          frame False {
            w3871 = 0 ("Column")
            n2993 = Decrement(x=w3870) -> (x-1=w3872:dbl)
            n2994 = Bundle By Name(cluster=w3867, "Row"=w3870, "Column"=w3871) -> (w3866:cluster{"Row":i32, "Column":i32})
            n2995 = Bundle By Name(cluster=w3866, "Row"=w3872, "Column"=w3871) -> (w3865:cluster{"Row":i32, "Column":i32})
            n2996 = property on="Step values" class="Tbl (strict)"("Active Cell"=w3865, "Cell BG Color"=u32 16711680 ("Active Cell:Cell Background Color")) -> ()  [unwired: 2 in, 2 out]
            n2997 = property on="Step values" class="Tbl (strict)"("Active Cell"=w3866, "Cell BG Color"=u32 16776072 ("Active Cell:Cell Background Color")) -> ()  [unwired: 2 in, 2 out]
          }
          frame True {
            n2998 = Bundle By Name(cluster=w3874, "Row"=w3876, "Column"=0) -> (w3873:cluster{"Row":i32, "Column":i32})
            n2999 = property on="Step values" class="Tbl (strict)"("Active Cell"=w3873, "Cell BG Color"=u32 16776072 ("Active Cell:Cell Background Color")) -> ()  [unwired: 2 in, 2 out]
          }
        }
        n3000 = call <vilib>:"Space Constant.vi"() -> ("String"=w3858:string)
        n3001 = Index Array(array=w3863, index (row)=w3864, index (col)=0 ("disabled index (col)")) -> (element=w3857:string)
        n3002 = call <vilib>:"Search and Replace Pattern.vi"("string"=w3857, "regular expression (\"\")"=w3858, "replace string (\"\")"="" ("replace string (\"\")"), "replace all? (F)"=TRUE) -> ("result string"=w3861:string)  [unwired: 1 in, 1 out]
        n3003 = Equal?(x="", y=w3861) -> (x = y?=w3859:bool)
        n3004 = Fract/Exp String To Number(string=w3861) -> (number=w3862:dbl)  [unwired: 3 in, 1 out]
        n3005 = case shown="False" w3859 {
          tunnel: w3862 -> [w3878 _]
          tunnel: w3851 -> [w3879 w4016]
          frame False {
            # "When step values are not finished"
            n3006 = property on="Current Step Value" class="DigNum (strict)"("Value"=w3878) -> ()  [unwired: 2 in, 2 out]
            n3007 = stacked-sequence {
              tunnel: w3878 -> [w3880 _ _]
              tunnel: w3879 -> [_ _ w4010]
              frame #0 {
                # "1 = 2400 1\n2 = 2400 2\n\n4 = 2636a smua\n5 = 2636a smub\n6 = do not sweep, just time\n7 = iPS, magnetic field \n8 = iTC, temperature"
                # "set next value in the sweep"
                n3008 = property on="step" class="RadioBtnsControl (strict)"() -> ("Value"=w3881:T2)  [unwired: 2 in, 2 out]
                n3009 = case shown="\"Radio Selection 8\"" w3881 {
                  tunnel: w3880 -> [w3883 w3890 _ _ _ _ _]
                  tunnel: w3880 -> [_ _ w3897 w3923 _ w3948 w3977]
                  frame "Radio Selection 1" {
                    # "sweep voltage on 2400 1"
                    n3010 = property on="2400_1_addr_step" class="DigNum (strict)"() -> ("Value"=w3882:u8)  [unwired: 2 in, 2 out]
                    n3011 = Number To Fractional String(number=w3883) -> (F-format string=w3888:string)  [unwired: 3 in]
                    n3012 = Concatenate Strings(":INIT:IMM; :SOUR:VOLT:LEV:IMM:AMPL " ("data"), w3888) -> (w3886:string)
                    n3013 = Number To Decimal String(number=w3882) -> (decimal integer string=w3884:string)  [unwired: 1 in]
                    n3014 = GPIB Write(0:w3884, 1:w3886, 2:i16 1 ("mode (0)")) -> ()  [unwired: 2 in, 2 out]
                  }
                  frame "Radio Selection 2" {
                    # "sweep voltage on 2400 2"
                    n3015 = property on="2400_2_addr_step" class="DigNum (strict)"() -> ("Value"=w3889:u8)  [unwired: 2 in, 2 out]
                    n3016 = Number To Fractional String(number=w3890) -> (F-format string=w3895:string)  [unwired: 3 in]
                    n3017 = Concatenate Strings(":INIT:IMM; :SOUR:CURR:LEV:IMM:AMPL " ("data"), w3895) -> (w3893:string)
                    n3018 = Number To Decimal String(number=w3889) -> (decimal integer string=w3891:string)  [unwired: 1 in]
                    n3019 = GPIB Write(0:w3891, 1:w3893, 2:i16 1 ("mode (0)")) -> ()  [unwired: 2 in, 2 out]
                  }
                  frame "Radio Selection 4" {
                    # "sweep voltage on 2636a smua"
                    n3020 = property on="Step Channel" class="DigNum (strict)"() -> ("Value"=w3899:dbl)  [unwired: 2 in, 2 out]
                    n3021 = property on="Mini steps" class="DigNum (strict)"() -> ("Value"=w3896:dbl)  [unwired: 2 in, 2 out]
